vi "FL_Last_N_Samples_Cluster_1D.vi"(1 "BufferLengthSamples":u32=100, 2 "Input 1D cluster array":T1(array[cluster])) -> (0 "Output 1D cluster array":T1(array[cluster]))   [LabVIEW 2018, in "Tracker.lvlib"]
uses:
  Tracker.lvlib
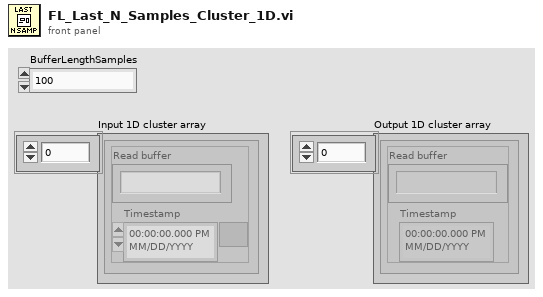
[diagram p1: front panel]
types:
  T1 = cluster{"Read buffer":string, "Timestamp":timestamp}[]
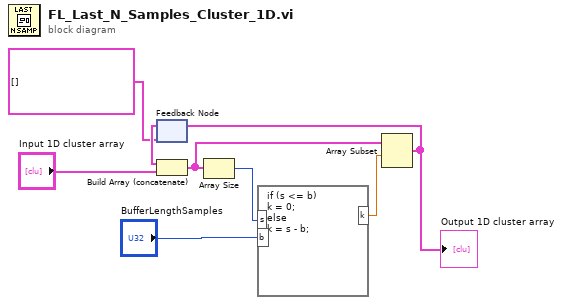
[diagram p0: block diagram]
diagram:
  n1 = feedback #1(T1 []) -> (w5:T1)
  n2 = Build Array (concatenate)(w5, "Input 1D cluster array") -> (w2:T1)
  n3 = Array Size(array=w2) -> (size(s)=w8:i32)
  n4 = formula code="if (s <= b)\nk = 0;\nelse\nk = s - b;"("s"=w8, "b"="BufferLengthSamples") -> ("k"=w7:dbl)
  n5 = Array Subset(array=w2, index=w7) -> (w1:T1)  [unwired: 1 in]
  "Output 1D cluster array" <- w1
  n6 = feedback-in #1(w1) -> ()
